vi "MH_WritePTUHeaderPostAcqV2.vi"(7 "FileOffset(bytes)":i64=3632, 8 "entrée d'erreur":errorcluster, 10 "TagArray":T1(array[cluster])=[{"TagIdent"="File_GUID", "TagIndex"=-1, "TagType"=1073872895, "TagValue"=40, "TagAuxData"="{197B8EE0-02FE-45EA-A6B5-3F8BBDE2D882}\u0000\u0000"}, {"TagIdent"="File_AssuredContent", "TagIndex"=-1, "TagType"=1073872895, "TagValue"=32, "TagAuxData"="MultiHarp: HWSETG SWSETG\u0000\u0000\u0000\u0000\u0000\u0000\u0000\u0000"}, {"TagIdent"="CreatorSW_ContentVersion", "TagIndex"=-1, "TagType"=1073872895, "TagValue"=8, "TagAuxData"="1.0\u0000\u0000\u0000\u0000\u0000"}, {"TagIdent"="CreatorSW_Name", "TagIndex"=-1, "TagType"=1073872895, "TagValue"=16, "TagAuxData"="MultiHarp AcqUI\u0000"}, {"TagIdent"="CreatorSW_Version", "TagIndex"=-1, "TagType"=1073872895, "TagValue"=8, "TagAuxData"="3.0.0.0\u0000"}, {"TagIdent"="File_CreatingTime", "TagIndex"=-1, "TagType"=553648136, "TagValue"=4676398420989345414, "TagAuxData"=""}, {"TagIdent"="File_Comment", "TagIndex"=-1, "TagType"=1073872895, "TagValue"=8, "TagAuxData"="T2 Mode\u0000"}, {"TagIdent"="Measurement_Mode", "TagIndex"=-1, "TagType"=268435464, "TagValue"=2, "TagAuxData"=""}, {"TagIdent"="Measurement_SubMode", "TagIndex"=-1, "TagType"=268435464, "TagValue"=0, "TagAuxData"=""}, {"TagIdent"="TTResult_StopReason", "TagIndex"=-1, "TagType"=268435464, "TagValue"=0, "TagAuxData"=""}, {"TagIdent"="Fast_Load_End", "TagIndex"=-1, "TagType"=-65528, "TagValue"=0, "TagAuxData"=""}, {"TagIdent"="TTResultFormat_TTTRRecType", "TagIndex"=-1, "TagType"=268435464, "TagValue"=66055, "TagAuxData"=""}, {"TagIdent"="TTResultFormat_BitsPerRecord", "TagIndex"=-1, "TagType"=268435464, "TagValue"=32, "TagAuxData"=""}, {"TagIdent"="MeasDesc_BinningFactor", "TagIndex"=-1, "TagType"=268435464, "TagValue"=32, "TagAuxData"=""}, {"TagIdent"="MeasDesc_Offset", "TagIndex"=-1, "TagType"=268435464, "TagValue"=0, "TagAuxData"=""}, {"TagIdent"="MeasDesc_AcquisitionTime", "TagIndex"=-1, "TagType"=268435464, "TagValue"=900000, "TagAuxData"=""}, {"TagIdent"="MeasDesc_StopAt", "TagIndex"=-1, "TagType"=268435464, "TagValue"=4294967295, "TagAuxData"=""}, {"TagIdent"="MeasDesc_StopOnOvfl", "TagIndex"=-1, "TagType"=8, "TagValue"=0, "TagAuxData"=""}, {"TagIdent"="MeasDesc_Restart", "TagIndex"=-1, "TagType"=8, "TagValue"=0, "TagAuxData"=""}, {"TagIdent"="CurSWSetting_DispLog", "TagIndex"=-1, "TagType"=8, "TagValue"=-1, "TagAuxData"=""}, {"TagIdent"="CurSWSetting_DispAxisTimeFrom", "TagIndex"=-1, "TagType"=268435464, "TagValue"=1, "TagAuxData"=""}, {"TagIdent"="CurSWSetting_DispAxisTimeTo", "TagIndex"=-1, "TagType"=268435464, "TagValue"=120, "TagAuxData"=""}, {"TagIdent"="CurSWSetting_DispAxisCountFrom", "TagIndex"=-1, "TagType"=268435464, "TagValue"=1, "TagAuxData"=""}, {"TagIdent"="CurSWSetting_DispAxisCountTo", "TagIndex"=-1, "TagType"=268435464, "TagValue"=10000, "TagAuxData"=""}, {"TagIdent"="CurSWSetting_DispCurves", "TagIndex"=-1, "TagType"=268435464, "TagValue"=16, "TagAuxData"=""}, {"TagIdent"="CurSWSetting_DispCurve_MapTo", "TagIndex"=0, "TagType"=268435464, "TagValue"=0, "TagAuxData"=""}, {"TagIdent"="CurSWSetting_DispCurve_Show", "TagIndex"=0, "TagType"=8, "TagValue"=-1, "TagAuxData"=""}, {"TagIdent"="CurSWSetting_DispCurve_MapTo", "TagIndex"=1, "TagType"=268435464, "TagValue"=1, "TagAuxData"=""}, {"TagIdent"="CurSWSetting_DispCurve_Show", "TagIndex"=1, "TagType"=8, "TagValue"=-1, "TagAuxData"=""}, {"TagIdent"="CurSWSetting_DispCurve_MapTo", "TagIndex"=2, "TagType"=268435464, "TagValue"=2, "TagAuxData"=""}, {"TagIdent"="CurSWSetting_DispCurve_Show", "TagIndex"=2, "TagType"=8, "TagValue"=-1, "TagAuxData"=""}, {"TagIdent"="CurSWSetting_DispCurve_MapTo", "TagIndex"=3, "TagType"=268435464, "TagValue"=3, "TagAuxData"=""}, {"TagIdent"="CurSWSetting_DispCurve_Show", "TagIndex"=3, "TagType"=8, "TagValue"=-1, "TagAuxData"=""}, {"TagIdent"="CurSWSetting_DispCurve_MapTo", "TagIndex"=4, "TagType"=268435464, "TagValue"=4, "TagAuxData"=""}, {"TagIdent"="CurSWSetting_DispCurve_Show", "TagIndex"=4, "TagType"=8, "TagValue"=-1, "TagAuxData"=""}, {"TagIdent"="CurSWSetting_DispCurve_MapTo", "TagIndex"=5, "TagType"=268435464, "TagValue"=5, "TagAuxData"=""}, {"TagIdent"="CurSWSetting_DispCurve_Show", "TagIndex"=5, "TagType"=8, "TagValue"=-1, "TagAuxData"=""}, {"TagIdent"="CurSWSetting_DispCurve_MapTo", "TagIndex"=6, "TagType"=268435464, "TagValue"=6, "TagAuxData"=""}, {"TagIdent"="CurSWSetting_DispCurve_Show", "TagIndex"=6, "TagType"=8, "TagValue"=-1, "TagAuxData"=""}, {"TagIdent"="CurSWSetting_DispCurve_MapTo", "TagIndex"=7, "TagType"=268435464, "TagValue"=7, "TagAuxData"=""}, {"TagIdent"="CurSWSetting_DispCurve_Show", "TagIndex"=7, "TagType"=8, "TagValue"=-1, "TagAuxData"=""}, {"TagIdent"="CurSWSetting_DispCurve_MapTo", "TagIndex"=8, "TagType"=268435464, "TagValue"=8, "TagAuxData"=""}, {"TagIdent"="CurSWSetting_DispCurve_Show", "TagIndex"=8, "TagType"=8, "TagValue"=-1, "TagAuxData"=""}, {"TagIdent"="CurSWSetting_DispCurve_MapTo", "TagIndex"=9, "TagType"=268435464, "TagValue"=9, "TagAuxData"=""}, {"TagIdent"="CurSWSetting_DispCurve_Show", "TagIndex"=9, "TagType"=8, "TagValue"=-1, "TagAuxData"=""}, {"TagIdent"="CurSWSetting_DispCurve_MapTo", "TagIndex"=10, "TagType"=268435464, "TagValue"=10, "TagAuxData"=""}, {"TagIdent"="CurSWSetting_DispCurve_Show", "TagIndex"=10, "TagType"=8, "TagValue"=-1, "TagAuxData"=""}, {"TagIdent"="CurSWSetting_DispCurve_MapTo", "TagIndex"=11, "TagType"=268435464, "TagValue"=11, "TagAuxData"=""}, {"TagIdent"="CurSWSetting_DispCurve_Show", "TagIndex"=11, "TagType"=8, "TagValue"=-1, "TagAuxData"=""}, {"TagIdent"="CurSWSetting_DispCurve_MapTo", "TagIndex"=12, "TagType"=268435464, "TagValue"=12, "TagAuxData"=""}, {"TagIdent"="CurSWSetting_DispCurve_Show", "TagIndex"=12, "TagType"=8, "TagValue"=-1, "TagAuxData"=""}, {"TagIdent"="CurSWSetting_DispCurve_MapTo", "TagIndex"=13, "TagType"=268435464, "TagValue"=13, "TagAuxData"=""}, {"TagIdent"="CurSWSetting_DispCurve_Show", "TagIndex"=13, "TagType"=8, "TagValue"=-1, "TagAuxData"=""}, {"TagIdent"="CurSWSetting_DispCurve_MapTo", "TagIndex"=14, "TagType"=268435464, "TagValue"=14, "TagAuxData"=""}, {"TagIdent"="CurSWSetting_DispCurve_Show", "TagIndex"=14, "TagType"=8, "TagValue"=-1, "TagAuxData"=""}, {"TagIdent"="CurSWSetting_DispCurve_MapTo", "TagIndex"=15, "TagType"=268435464, "TagValue"=15, "TagAuxData"=""}, {"TagIdent"="CurSWSetting_DispCurve_Show", "TagIndex"=15, "TagType"=8, "TagValue"=-1, "TagAuxData"=""}, {"TagIdent"="HW_Type", "TagIndex"=-1, "TagType"=1073872895, "TagValue"=24, "TagAuxData"="MultiHarp 150 4P\u0000\u0000\u0000\u0000\u0000\u0000\u0000\u0000"}, {"TagIdent"="HW_PartNo", "TagIndex"=-1, "TagType"=1073872895, "TagValue"=8, "TagAuxData"="930043\u0000\u0000"}, {"TagIdent"="HW_Version", "TagIndex"=-1, "TagType"=1073872895, "TagValue"=8, "TagAuxData"="1.0\u0000\u0000\u0000\u0000\u0000"}, {"TagIdent"="HW_SerialNo", "TagIndex"=-1, "TagType"=1073872895, "TagValue"=8, "TagAuxData"="1043897\u0000"}, {"TagIdent"="HW_Features", "TagIndex"=-1, "TagType"=285212680, "TagValue"=183, "TagAuxData"=""}, {"TagIdent"="HW_BaseResolution", "TagIndex"=-1, "TagType"=536870920, "TagValue"=4437731733528994965, "TagAuxData"=""}, {"TagIdent"="HW_InpChannels", "TagIndex"=-1, "TagType"=268435464, "TagValue"=4, "TagAuxData"=""}, {"TagIdent"="HW_ExternalRefClock", "TagIndex"=-1, "TagType"=8, "TagValue"=0, "TagAuxData"=""}, {"TagIdent"="HW_ExternalDevices", "TagIndex"=-1, "TagType"=268435464, "TagValue"=0, "TagAuxData"=""}, {"TagIdent"="HWTriggerOut_Period", "TagIndex"=-1, "TagType"=536870920, "TagValue"=4502148214488346441, "TagAuxData"=""}, {"TagIdent"="HWTriggerOut_On", "TagIndex"=-1, "TagType"=8, "TagValue"=0, "TagAuxData"=""}, {"TagIdent"="HW_InputHysteresis", "TagIndex"=-1, "TagType"=8, "TagValue"=0, "TagAuxData"=""}, {"TagIdent"="HWSync_Divider", "TagIndex"=-1, "TagType"=268435464, "TagValue"=1, "TagAuxData"=""}, {"TagIdent"="HWSync_TrgLevel", "TagIndex"=-1, "TagType"=268435464, "TagValue"=-10, "TagAuxData"=""}, {"TagIdent"="HWSync_TrgEdge", "TagIndex"=-1, "TagType"=268435464, "TagValue"=0, "TagAuxData"=""}, {"TagIdent"="HWSync_Offset", "TagIndex"=-1, "TagType"=268435464, "TagValue"=27000, "TagAuxData"=""}, {"TagIdent"="HWSync_TdCode", "TagIndex"=-1, "TagType"=268435464, "TagValue"=0, "TagAuxData"=""}, {"TagIdent"="HWInpChan_TrgLevel", "TagIndex"=0, "TagType"=268435464, "TagValue"=-150, "TagAuxData"=""}, {"TagIdent"="HWInpChan_TrgEdge", "TagIndex"=0, "TagType"=268435464, "TagValue"=0, "TagAuxData"=""}, {"TagIdent"="HWInpChan_Offset", "TagIndex"=0, "TagType"=268435464, "TagValue"=0, "TagAuxData"=""}, {"TagIdent"="HWInpChan_Enabled", "TagIndex"=0, "TagType"=8, "TagValue"=-1, "TagAuxData"=""}, {"TagIdent"="HWInpChan_TdCode", "TagIndex"=0, "TagType"=268435464, "TagValue"=0, "TagAuxData"=""}, {"TagIdent"="HWInpChan_TrgLevel", "TagIndex"=1, "TagType"=268435464, "TagValue"=-150, "TagAuxData"=""}, {"TagIdent"="HWInpChan_TrgEdge", "TagIndex"=1, "TagType"=268435464, "TagValue"=0, "TagAuxData"=""}, {"TagIdent"="HWInpChan_Offset", "TagIndex"=1, "TagType"=268435464, "TagValue"=0, "TagAuxData"=""}, {"TagIdent"="HWInpChan_Enabled", "TagIndex"=1, "TagType"=8, "TagValue"=-1, "TagAuxData"=""}, {"TagIdent"="HWInpChan_TdCode", "TagIndex"=1, "TagType"=268435464, "TagValue"=0, "TagAuxData"=""}, {"TagIdent"="HWInpChan_TrgLevel", "TagIndex"=2, "TagType"=268435464, "TagValue"=-50, "TagAuxData"=""}, {"TagIdent"="HWInpChan_TrgEdge", "TagIndex"=2, "TagType"=268435464, "TagValue"=0, "TagAuxData"=""}, {"TagIdent"="HWInpChan_Offset", "TagIndex"=2, "TagType"=268435464, "TagValue"=0, "TagAuxData"=""}, {"TagIdent"="HWInpChan_Enabled", "TagIndex"=2, "TagType"=8, "TagValue"=-1, "TagAuxData"=""}, {"TagIdent"="HWInpChan_TdCode", "TagIndex"=2, "TagType"=268435464, "TagValue"=0, "TagAuxData"=""}, {"TagIdent"="HWInpChan_TrgLevel", "TagIndex"=3, "TagType"=268435464, "TagValue"=-50, "TagAuxData"=""}, {"TagIdent"="HWInpChan_TrgEdge", "TagIndex"=3, "TagType"=268435464, "TagValue"=0, "TagAuxData"=""}, {"TagIdent"="HWInpChan_Offset", "TagIndex"=3, "TagType"=268435464, "TagValue"=0, "TagAuxData"=""}, {"TagIdent"="HWInpChan_Enabled", "TagIndex"=3, "TagType"=8, "TagValue"=-1, "TagAuxData"=""}, {"TagIdent"="HWInpChan_TdCode", "TagIndex"=3, "TagType"=268435464, "TagValue"=0, "TagAuxData"=""}, {"TagIdent"="MeasDesc_Resolution", "TagIndex"=-1, "TagType"=536870920, "TagValue"=4437731733528994965, "TagAuxData"=""}, {"TagIdent"="HW_Markers", "TagIndex"=-1, "TagType"=268435464, "TagValue"=4, "TagAuxData"=""}, {"TagIdent"="HWMarkers_RisingEdge", "TagIndex"=0, "TagType"=8, "TagValue"=0, "TagAuxData"=""}, {"TagIdent"="HWMarkers_RisingEdge", "TagIndex"=1, "TagType"=8, "TagValue"=0, "TagAuxData"=""}, {"TagIdent"="HWMarkers_RisingEdge", "TagIndex"=2, "TagType"=8, "TagValue"=0, "TagAuxData"=""}, {"TagIdent"="HWMarkers_RisingEdge", "TagIndex"=3, "TagType"=8, "TagValue"=0, "TagAuxData"=""}, {"TagIdent"="HWMarkers_Enabled", "TagIndex"=0, "TagType"=8, "TagValue"=-1, "TagAuxData"=""}, {"TagIdent"="HWMarkers_Enabled", "TagIndex"=1, "TagType"=8, "TagValue"=-1, "TagAuxData"=""}, {"TagIdent"="HWMarkers_Enabled", "TagIndex"=2, "TagType"=8, "TagValue"=-1, "TagAuxData"=""}, {"TagIdent"="HWMarkers_Enabled", "TagIndex"=3, "TagType"=8, "TagValue"=-1, "TagAuxData"=""}, {"TagIdent"="HWMarkers_HoldOff", "TagIndex"=-1, "TagType"=268435464, "TagValue"=0, "TagAuxData"=""}, {"TagIdent"="MeasDesc_GlobalResolution", "TagIndex"=-1, "TagType"=536870920, "TagValue"=4437731733528994965, "TagAuxData"=""}, {"TagIdent"="TTResult_SyncRate", "TagIndex"=-1, "TagType"=268435464, "TagValue"=0, "TagAuxData"=""}, {"TagIdent"="TTResult_InputRate", "TagIndex"=0, "TagType"=268435464, "TagValue"=9126, "TagAuxData"=""}, {"TagIdent"="TTResult_InputRate", "TagIndex"=1, "TagType"=268435464, "TagValue"=8247, "TagAuxData"=""}, {"TagIdent"="TTResult_InputRate", "TagIndex"=2, "TagType"=268435464, "TagValue"=0, "TagAuxData"=""}, {"TagIdent"="TTResult_InputRate", "TagIndex"=3, "TagType"=268435464, "TagValue"=0, "TagAuxData"=""}, {"TagIdent"="TTResult_StopAfter", "TagIndex"=-1, "TagType"=268435464, "TagValue"=900000, "TagAuxData"=""}, {"TagIdent"="TTResult_NumberOfRecords", "TagIndex"=-1, "TagType"=268435464, "TagValue"=10000, "TagAuxData"=""}, {"TagIdent"="TTResult_MDescWarningFlags", "TagIndex"=-1, "TagType"=285212680, "TagValue"=0, "TagAuxData"=""}, {"TagIdent"="Header_End", "TagIndex"=-1, "TagType"=-65528, "TagValue"=0, "TagAuxData"=""}], 11 "refnum In":refnum<file>) -> (0 "sortie d'erreur":errorcluster, 3 "refnum Out":refnum<file>)   [LabVIEW 2019]
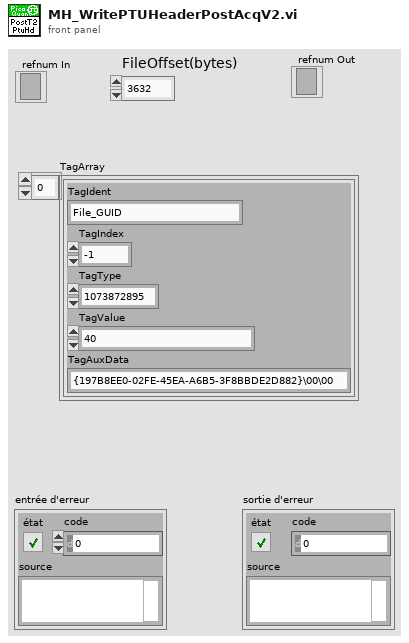
[diagram p1: front panel]
types:
  T1 = cluster{"TagIdent":string, "TagIndex":i32, "TagType":i32, "TagValue":i64, "TagAuxData":string}[]
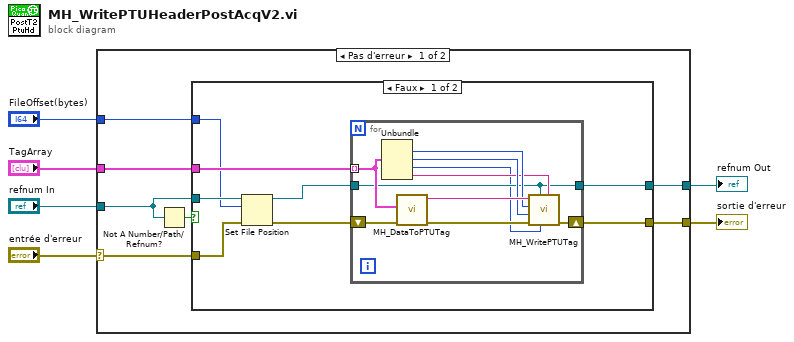
[diagram p0: block diagram]
diagram:
  n1 = case shown="Pas d'erreur" "entrée d'erreur" {
    selector: "entrée d'erreur" -> [w7 w34]
    tunnel: [w13 w34] -> w6
    tunnel: "refnum In" -> [w8 _]
    tunnel: "TagArray" -> [w12 _]
    tunnel: [w11 _] -> w3
    tunnel: "FileOffset(bytes)" -> [w9 _]
    frame No Error {
      n2 = Not A Number/Path/Refnum?(number/path/refnum=w8) -> (NaN/Path/Refnum?=w10:bool)
      n3 = case shown="Faux" w10 {
        tunnel: w7 -> [w19 w33]
        tunnel: [w14 w33] -> w13
        tunnel: w8 -> [w17 w32]
        tunnel: w12 -> [w21 _]
        tunnel: [w20 w32] -> w11
        tunnel: w9 -> [w15 _]
        frame False {
          n4 = Set File Position(offset (in bytes) (0)=w15, refnum=w17, error in=w19) -> (refnum out=w16:refnum<file>, error out=w18:errorcluster)  [unwired: 1 in]
          n5 = for {
            tunnel: w21 -> [w31] mode=indexing
            shift-right: [w24] -> w14
            shift-left: w18 -> [w25]
            tunnel: w16 -> [w23]
            tunnel: [w23] -> w20
            n6 = Unbundle(w31) -> ("TagIndex"=w29:i32, "TagType"=w28:i32, "TagValue"=w22:i64, "TagAuxData"=w27:string)  [unwired: 1 out]
            n7 = call <userlib>:"MH_DataToPTUTag.vi"("error in"=w25, "TagIn"=w31) -> ("error in 2"=w26:errorcluster, "TagIdent Out"=w30:string)  [unwired: 5 in, 3 out]
            n8 = call <userlib>:"MH_WritePTUTag.vi"("TagAuxData"=w27, "TagValue"=w22, "refnum"=w23, "error in"=w26, "TagType"=w28, "TagIndex"=w29, "identifierfull"=w30) -> ("error out"=w24:errorcluster)  [unwired: 3 in]
          }
        }
        frame True {
        }
      }
    }
    frame Error {
    }
  }
  "sortie d'erreur" <- w6
  "refnum Out" <- w3
